vi "PicohrdlGetSingleValueAsync.vi"(8 "error in (no error)":errorcluster, 11 "handle in":i16) -> (0 "error out":errorcluster, 1 "value":i32, 3 "Handle out":i16, 4 "Over Voltage":i16)   [LabVIEW 2010]
doc: "Calls HRDLGetSingleValueAsync()"
uses:
  PicoHRDL.dll
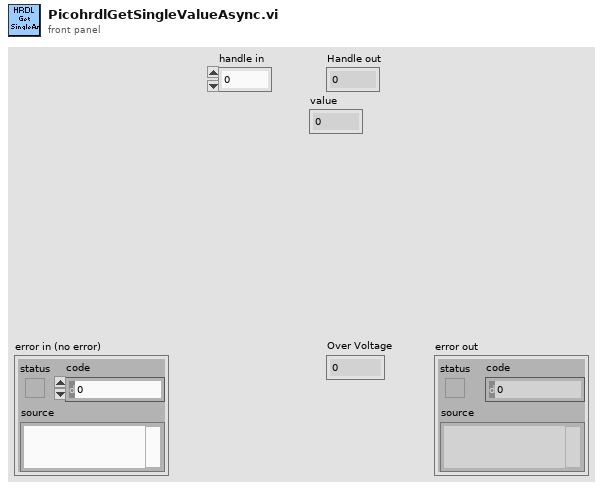
[diagram p1: front panel]
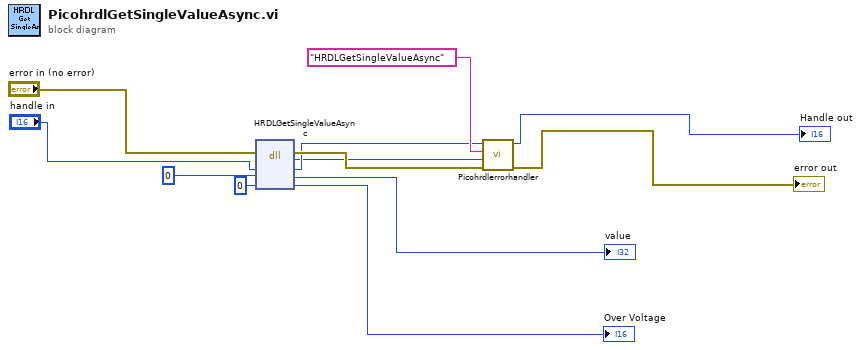
[diagram p0: block diagram]
diagram:
  n1 = dll-call lib="PicoHRDL.dll" fn="HRDLGetSingleValueAsync"(error in="error in (no error)", "handle"="handle in", "value"=0, "overflow"=i16 0) -> (error out=w5:errorcluster, "return type"=w3:i16, "handle"=w4:i16, "value"=→"value":i32, "overflow"=→"Over Voltage":i16)  [unwired: 2 in, 1 out]
  n2 = call "Picohrdlerrorhandler.vi"("Handle in"=w4, "API function"="HRDLGetSingleValueAsync", "Return"=w3, "error in (no error)"=w5) -> ("Handle out"=→"Handle out":i16, "error out"=→"error out":errorcluster)  [unwired: 5 in]
